vi "header_out.vi"(10 "FINS Header":T1={"resp req"=TRUE, "cmd resp"=FALSE, "SID"=0, "DNA"=0, "DA1"=10, "DA2"=0, "SA1"=251, "SA2"=0, "SNA"=255} {"SNA" max=127 format="%x"; "SA2" max=254 step=1 format="%x"; "SA1" format="%x"; "DA2" max=254 step=1 format="%x"; "DA1" format="%x"; "DNA" max=127 step=1 format="%x"}) -> (2 "FINS Header":string)   [LabVIEW 2019, in "FINS TCP.lvlib"]
uses:
  FINS TCP.lvlib
  FINS_header.ctl
panel:
  out "Numeric":u8=129 format="%b"
  out "length":i32=10
  out "output array":u8[](array[numeric])=[129, 0, 2, 10, 0, 0, 255, 255, 255, 255] format="%b"
  # "1.ICS"
  # "2.RSV"
  # "3.GCT"
  # "4.DNA"
  # "5.DA1"
  # "6.DA2"
  # "7.SNA"
  # "8.SA1_node"
  # "9.SA1_unit"
  # "10.SID"
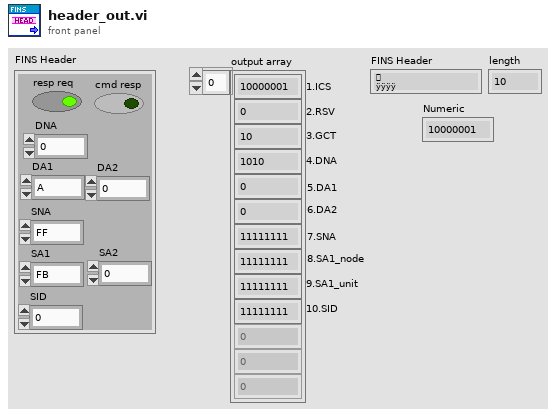
[diagram p1: front panel]
types:
  T1 = typedef "FINS TCP.lvlib/FINS_header.ctl" = cluster{"resp req":bool, "cmd resp":bool, "SID":u8, "DNA":u8, "DA1":u8, "DA2":u8, "SA1":u8, "SA2":u8, "SNA":u8}
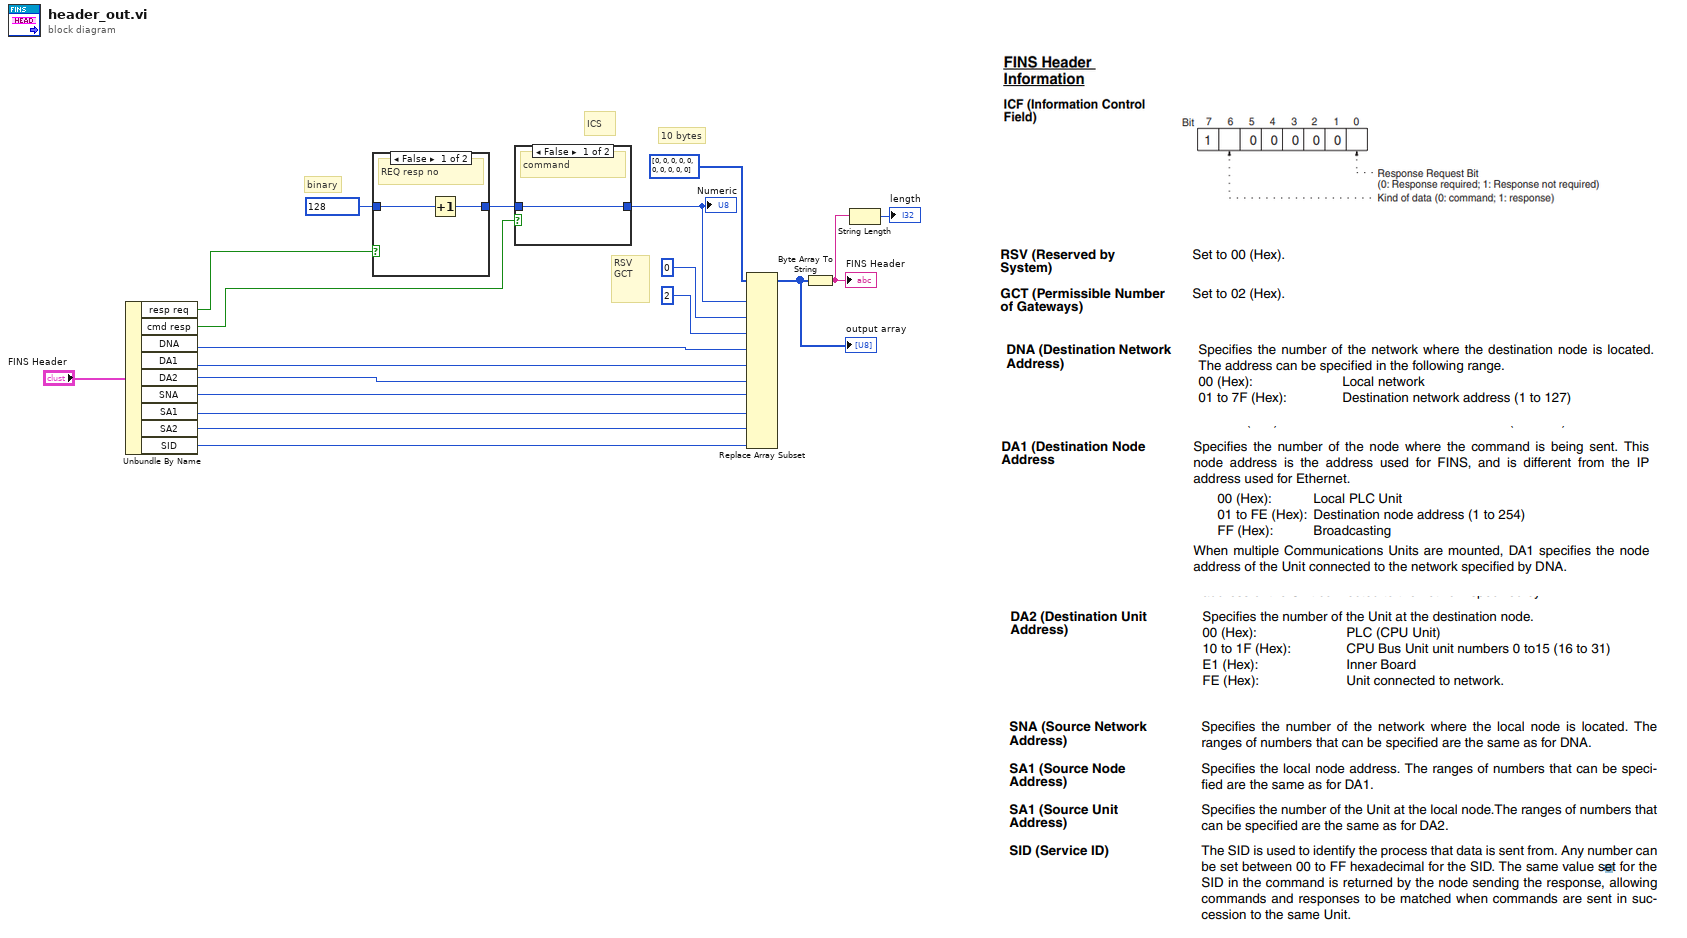
[diagram p0: block diagram]
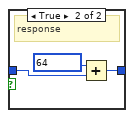
[diagram p2: hidden frame]
diagram:
  # "binary"
  # "10 bytes"
  # "RSV\nGCT"
  # "ICS"
  n1 = Unbundle By Name("FINS Header") -> ("resp req"=w8:bool, "cmd resp"=w7:bool, "DNA"=w10:u8, "DA1"=w9:u8, "DA2"=w4:u8, "SNA"=w3:u8, "SA1"=w2:u8, "SA2"=w1:u8, "SID"=w11:u8)
  n2 = case shown="False" w8 {
    tunnel: u8 128 -> [w21 w22]
    tunnel: [w20 w22] -> w18
    frame False {
      # "REQ resp no"
      n3 = Increment(x=w21) -> (x+1=w20:u8)
    }
    frame True {
      # "REQ resp yes"
    }
  }
  n4 = case shown="False" w7 {
    tunnel: w18 -> [w23 w26]
    tunnel: [w23 w25] -> w16
    frame False {
      # "command"
    }
    frame True {
      # "response"
      n5 = Add(x=u8 64, y=w26) -> (x+y=w25:u8)
    }
  }
  "Numeric" <- w16
  n6 = Replace Array Subset(array=u8[] [0, 0, 0, 0, 0, 0, 0, 0, 0, 0], new element #1=w16, new element #2=u8 0, new element #3=u8 2, new element #4=w10, new element #5=w9, new element #6=w4, new element #7=w3, new element #8=w2, new element #9=w1, new element #10=w11) -> (w13:u8[])  [unwired: 10 in]
  "output array" <- w13
  n7 = Byte Array To String(unsigned byte array=w13) -> (string=w6:string)
  "FINS Header" <- w6
  n8 = String Length(string=w6) -> (length=→"length":i32)
